vi "Mem4.vi"(4 "Phi1":bool, 6 "Phi0":bool, 11 "Data In":bool) -> (3 "Data Out":bool)   [LabVIEW 2012]
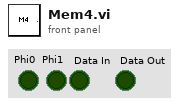
[diagram p1: front panel]
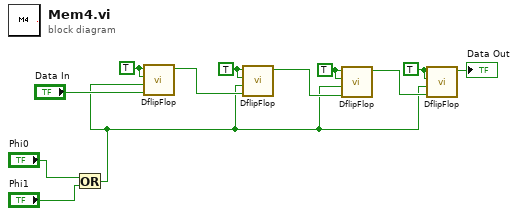
[diagram p0: block diagram]
diagram:
  w6 = TRUE ("Set")
  w8 = TRUE ("Set")
  w10 = TRUE ("Set")
  w12 = TRUE ("Set")
  n1 = Or(x="Phi0", y="Phi1") -> (x .or. y?=w1:bool)
  n2 = call "DflipFlop.vi"("D"="Data In", "Clock"=w1, "Reset"=w12, "Set"=w12) -> ("Q"=w11:bool)  [unwired: 6 in, 1 out]
  n3 = call "DflipFlop.vi"("D"=w11, "Clock"=w1, "Reset"=w10, "Set"=w10) -> ("Q"=w9:bool)  [unwired: 6 in, 1 out]
  n4 = call "DflipFlop.vi"("D"=w9, "Clock"=w1, "Reset"=w8, "Set"=w8) -> ("Q"=w7:bool)  [unwired: 6 in, 1 out]
  n5 = call "DflipFlop.vi"("D"=w7, "Clock"=w1, "Reset"=w6, "Set"=w6) -> ("Q"=→"Data Out":bool)  [unwired: 6 in, 1 out]
